vi "ArthOps.vi"() -> ()   [LabVIEW 2026]
panel:
  out "1/x":dbl
  out "x+y":dbl
  out "x*y":dbl
  out "x-1":dbl
  out "x*2^n":dbl
  in  "x":dbl
  in  "y":dbl
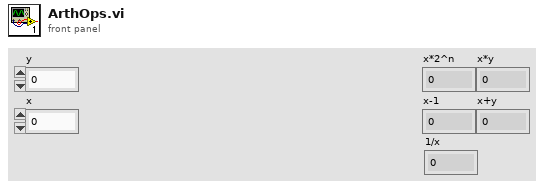
[diagram p1: front panel]
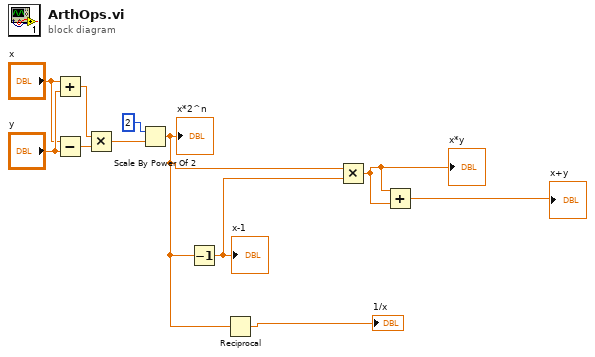
[diagram p0: block diagram]
diagram:
  n1 = Add(x="x", y="y") -> (x+y=w9:dbl)
  n2 = Subtract(x="x", y="y") -> (x-y=w8:dbl)
  n3 = Multiply(x=w9, y=w8) -> (x*y=w7:dbl)
  n4 = Scale By Power Of 2(n=i16 2, x=w7) -> (x*2^n=w2:dbl)
  "x*2^n" <- w2
  n5 = Decrement(x=w2) -> (x-1=w5:dbl)
  "x-1" <- w5
  n6 = Reciprocal(x=w2) -> (1/x=→"1/x":dbl)
  n7 = Multiply(x=w2, y=w5) -> (x*y=w4:dbl)
  "x*y" <- w4
  n8 = Add(x=w4, y=w4) -> (x+y=→"x+y":dbl)
